vi "SendExitEvent.vi"(8 "error in (no error)":errorcluster, 11 "ByRefClass in":refnum<class "ClassByRef.lvclass">) -> (0 "error out":errorcluster, 3 "ByRefClass out":refnum<class "ClassByRef.lvclass">)   [LabVIEW 2021, in "ClassUtilities.lvlib" / "ClassByRef.lvclass"]
uses:
  ClassByRef.lvclass
  <vilib>/event_ctls.llb/usereventprio.ctl
  ClassByRef.lvclass/ClassByRef.ctl
  GetExitEvent.vi
  GetExitEvent.vi/d78f5ac1-b881-48f7-a86d-8a9fda2b8e49.vi
  GetRef.vi
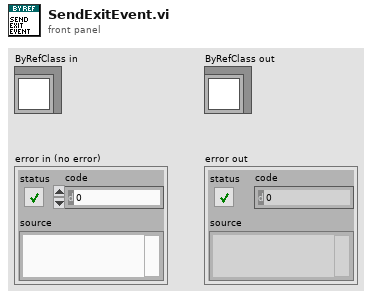
[diagram p1: front panel]
types:
  T1 = typedef "usereventprio.ctl" = enum32{"high priority", "normal priority"}
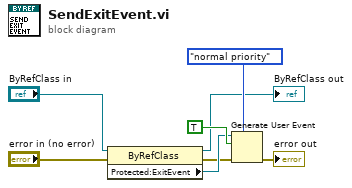
[diagram p0: block diagram]
diagram:
  n1 = property class="ByRefClass"(reference="ByRefClass in", error in="error in (no error)") -> (reference out=→"ByRefClass out":refnum<class "ClassByRef.lvclass">, error out=w2:errorcluster, "Protected:ExitEvent"=w3:refnum<user-event>)
  n2 = Generate User Event(priority (normal)=usereventprio."normal priority", user event=w3, event data cluster=TRUE ("event data"), error in=w2) -> (error out=→"error out":errorcluster)  [unwired: 1 out]
